vi "Cluster Get Datatype.vi"(8 "Error In":errorcluster, 11 "cluster variant in":variant) -> (0 "Error Out":errorcluster, 3 "cluster datatype":string)   [LabVIEW 2018]
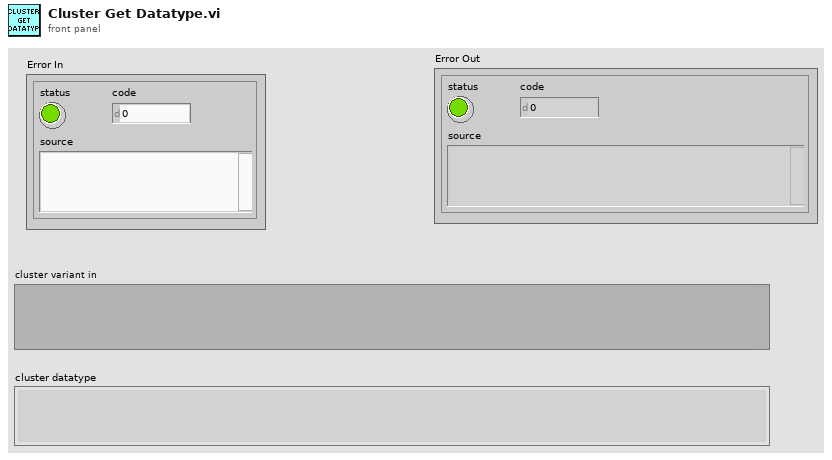
[diagram p1: front panel]
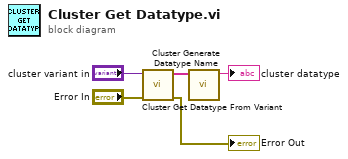
[diagram p0: block diagram]
diagram:
  n1 = call "Cluster Get Datatype From Variant.vi"("Error In"="Error In", "cluster variant in"="cluster variant in") -> ("Error Out"=→"Error Out":errorcluster, "cluster elements datatypes"=w5:string[])  [unwired: 8 in]
  n2 = call "Cluster Generate Datatype Name.vi"("Cluster elements datatypes"=w5) -> ("generated datatype name"=→"cluster datatype":string)  [unwired: 10 in]
